vi "LTVUnicycleCtrl_Execute.vi"(4 "dT Sec":dbl=0.02, 5 "LTV_Unicycle_Ctrl_Model":T2={"Max linear ctrl effort M/S"=1.0, "Max angular ctrl effort Rad/S"=2.0, "Max Heading Meas Tol Rad"=0.2, "Max X Pos Meas Tol M"=0.0625, "Max Y Pos Meas Tol M"=0.125, "Max Linear Vel M/S"=9.0} {"Max Linear Vel M/S" format="%#_13g"; "Max Y Pos Meas Tol M" format="%#_13g"; "Max X Pos Meas Tol M" format="%#_13g"; "Max Heading Meas Tol Rad" format="%#_13g"; "Max angular ctrl effort Rad/S" format="%#_13g"; "Max linear ctrl effort M/S" format="%#_13g"}, 6 "Enabled":bool=TRUE, 7 "LTV_Unicycle_Ctrl_Tolerance":T1={"Max Heading Tolerance Rad"=1.0, "Max X Tolerance M"=2.0, "Max Y Tolerance M"=0.2} {"Max Y Tolerance M" format="%#_13g"; "Max X Tolerance M" format="%#_13g"; "Max Heading Tolerance Rad" format="%#_13g"}, 8 "CurrentPose":T4={"TRANSLATION"={"X"=0.0, "Y"=0.0}, "ROTATION"={"VALUE"=0.0, "COS"=1.0, "SIN"=0.0}} {"ROTATION"."SIN" format="%13.4f"; "ROTATION"."COS" format="%13.4f"; "ROTATION"."VALUE" format="%13.4f"; "TRANSLATION"."Y" format="%14.3f"; "TRANSLATION"."X" format="%14.3f"}, 9 "RefAngularVelocity":dbl, 10 "RefLinearVelocity":dbl, 11 "RefPose":T4={"TRANSLATION"={"X"=0.0, "Y"=0.0}, "ROTATION"={"VALUE"=0.0, "COS"=1.0, "SIN"=0.0}} {"ROTATION"."SIN" format="%13.4f"; "ROTATION"."COS" format="%13.4f"; "ROTATION"."VALUE" format="%13.4f"; "TRANSLATION"."Y" format="%14.3f"; "TRANSLATION"."X" format="%14.3f"}) -> (0 "Error":bool, 1 "out LTV_UNICYCLE_CONTROLLER":T7={"States"=0, "Inputs"=0, "PoseError"={"TRANSLATION"={"X"=0.0, "Y"=0.0}, "ROTATION"={"VALUE"=0.0, "COS"=1.0, "SIN"=0.0}}, "PoseTolerance"={"TRANSLATION"={"X"=0.0, "Y"=0.0}, "ROTATION"={"VALUE"=0.0, "COS"=1.0, "SIN"=0.0}}, "Dt"=0.02, "Enabled"=FALSE, "LQR_K_Table"={"Table Xs"=[], "Table Ys"=[], "MinX"=0.0, "MaxX"=0.0, "ItemCount"=0, "Rows"=0, "Columns"=0}} {"PoseTolerance"."ROTATION"."SIN" format="%13.4f"; "PoseTolerance"."ROTATION"."COS" format="%13.4f"; "PoseTolerance"."ROTATION"."VALUE" format="%13.4f"; "PoseTolerance"."TRANSLATION"."Y" format="%14.3f"; "PoseTolerance"."TRANSLATION"."X" format="%14.3f"; "PoseError"."ROTATION"."SIN" format="%13.4f"; "PoseError"."ROTATION"."COS" format="%13.4f"; "PoseError"."ROTATION"."VALUE" format="%13.4f"; "PoseError"."TRANSLATION"."Y" format="%14.3f"; "PoseError"."TRANSLATION"."X" format="%14.3f"}, 2 "At Reference":bool, 3 "ChassisSpeeds":T3 {"vOmega" format="%10.3f"; "vY" format="%10.3f"; "vX" format="%10.3f"})   [LabVIEW 2019, in "Trajectory_Library.lvlib"]
doc: "The linear time-varying unicycle controller has a similar form to the LQR, but the model used to compute the controller gain is the nonlinear model linearized around the drivetrain's current state.\n\nThis LabVIEW single call function creates and executes the LTV Unicycle controller. \n\n\nInputs:\n - LTVUnicycleCtrl Model -- cluster -- Packed data used to construct the LTV Unicycle control system.\n - LTVUnicycleCtrl Tol -- cluster -- Packed data used to define the tolerance LTV Unicycle control system.\n - Ref Pose -- Pose2d -- The desired pose setpoint. (Meters, Radians)\n - Ref Linear Velocity -- double -- The desired linear velocity (Meters/sec)\n - Ref Angular Velocity -- double -- The desired angular velocity (Radians/sec)\n - Current Pose -- Pose2d -- The current pose. (Meters, Radians)\n - Enabled -- boolean -- If TRUE use closed loop control to calculate desired chassis speeds. If FALSE, outputs the reference speeds directly.\n - dt Sec -- double -- Update time (default: 0.02)\n\nOutputs:\n - Chassis Speed -- chassis speed -- Chassis Speed Demand\n - At Reference -- boolean -- If TRUE, the current position is within the tolerance.\n - Error -- boolean -- If TRUE, an error occured.\n - out LTV UnicycleCtrl -- cluster -- Internal data structure."
uses:
  Trajectory_Library.lvlib
  TypeDef/LTV_UNICYCLE_CONTROLLER.ctl
  TypeDef/POSE2D.ctl
  TypeDef/TRANSLATION2D.ctl
  TypeDef/ROTATION2D.ctl
  TypeDef/FUNCTION_GENERATOR_MATRIX.ctl
  TypeDef/CHASSIS_SPEEDS.ctl
  TypeDef/LTV_UNICYCLE_CONTROLLER_MODEL_PARAMS.CTL
  TypeDef/LTV_UNICYCLE_CONTROLLER_TOLERANCE.CTL
  Rotation2d_CreateAngle.vi
  Translation2d_Create.vi
  MatBuilder_Create.vi
  Pose2d_getXYAngle.vi
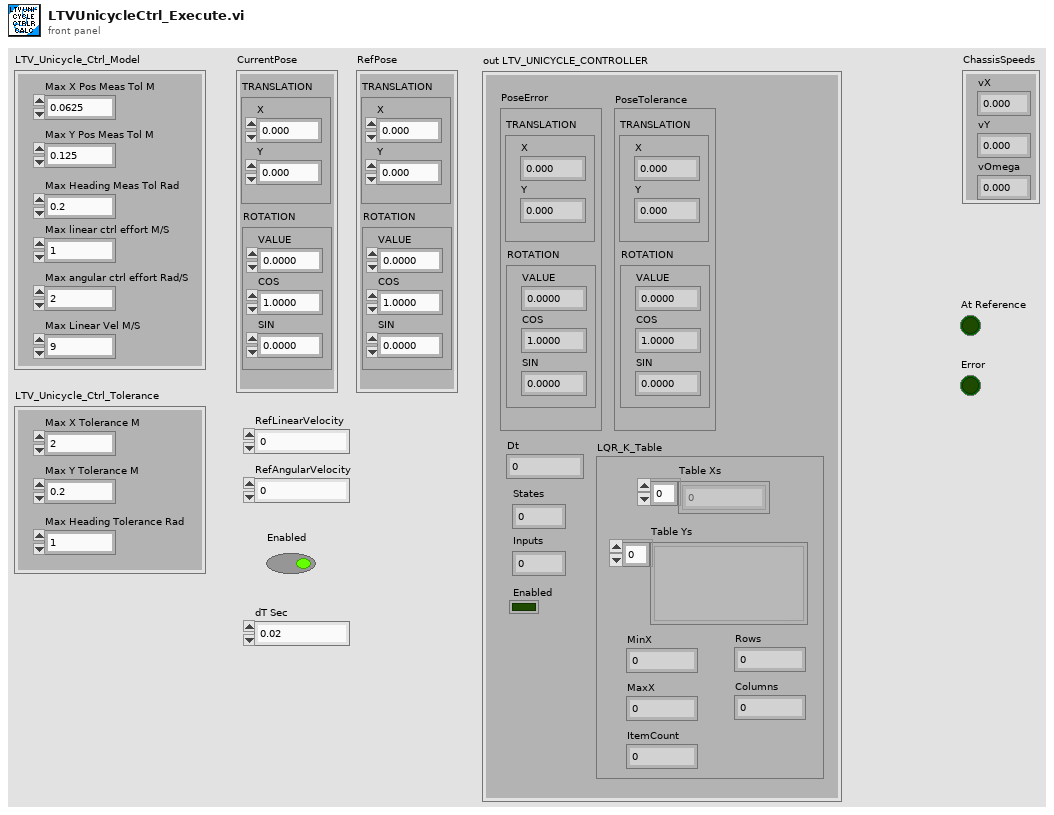
[diagram p1: front panel]
types:
  T1 = typedef "Trajectory_Library.lvlib/LTV_UNICYCLE_CONTROLLER_TOLERANCE.CTL" = cluster{"Max Heading Tolerance Rad":dbl, "Max X Tolerance M":dbl, "Max Y Tolerance M":dbl}
  T2 = typedef "Trajectory_Library.lvlib/LTV_UNICYCLE_CONTROLLER_MODEL_PARAMS.CTL" = cluster{"Max linear ctrl effort M/S":dbl, "Max angular ctrl effort Rad/S":dbl, "Max Heading Meas Tol Rad":dbl, "Max X Pos Meas Tol M":dbl, "Max Y Pos Meas Tol M":dbl, "Max Linear Vel M/S":dbl}
  T3 = typedef "Trajectory_Library.lvlib/CHASSIS_SPEEDS.ctl" = cluster{"vX":dbl, "vY":dbl, "vOmega":dbl}
  T4 = typedef "Trajectory_Library.lvlib/POSE2D.ctl" = cluster{"TRANSLATION":T5, "ROTATION":T6}
  T5 = typedef "Trajectory_Library.lvlib/TRANSLATION2D.ctl" = cluster{"X":dbl, "Y":dbl}
  T6 = typedef "Trajectory_Library.lvlib/ROTATION2D.ctl" = cluster{"VALUE":dbl, "COS":dbl, "SIN":dbl}
  T7 = typedef "Trajectory_Library.lvlib/LTV_UNICYCLE_CONTROLLER.ctl" = cluster{"States":i32, "Inputs":i32, "PoseError":T4, "PoseTolerance":T4, "Dt":dbl, "Enabled":bool, "LQR_K_Table":T8}
  T8 = typedef "Trajectory_Library.lvlib/FUNCTION_GENERATOR_MATRIX.ctl" = cluster{"Table Xs":dbl[], "Table Ys":variant[], "MinX":dbl, "MaxX":dbl, "ItemCount":i32, "Rows":i32, "Columns":i32}
  T9 = typedef "NI_Matrix.lvlib/RealMatrix.ctl" = dbl[][]
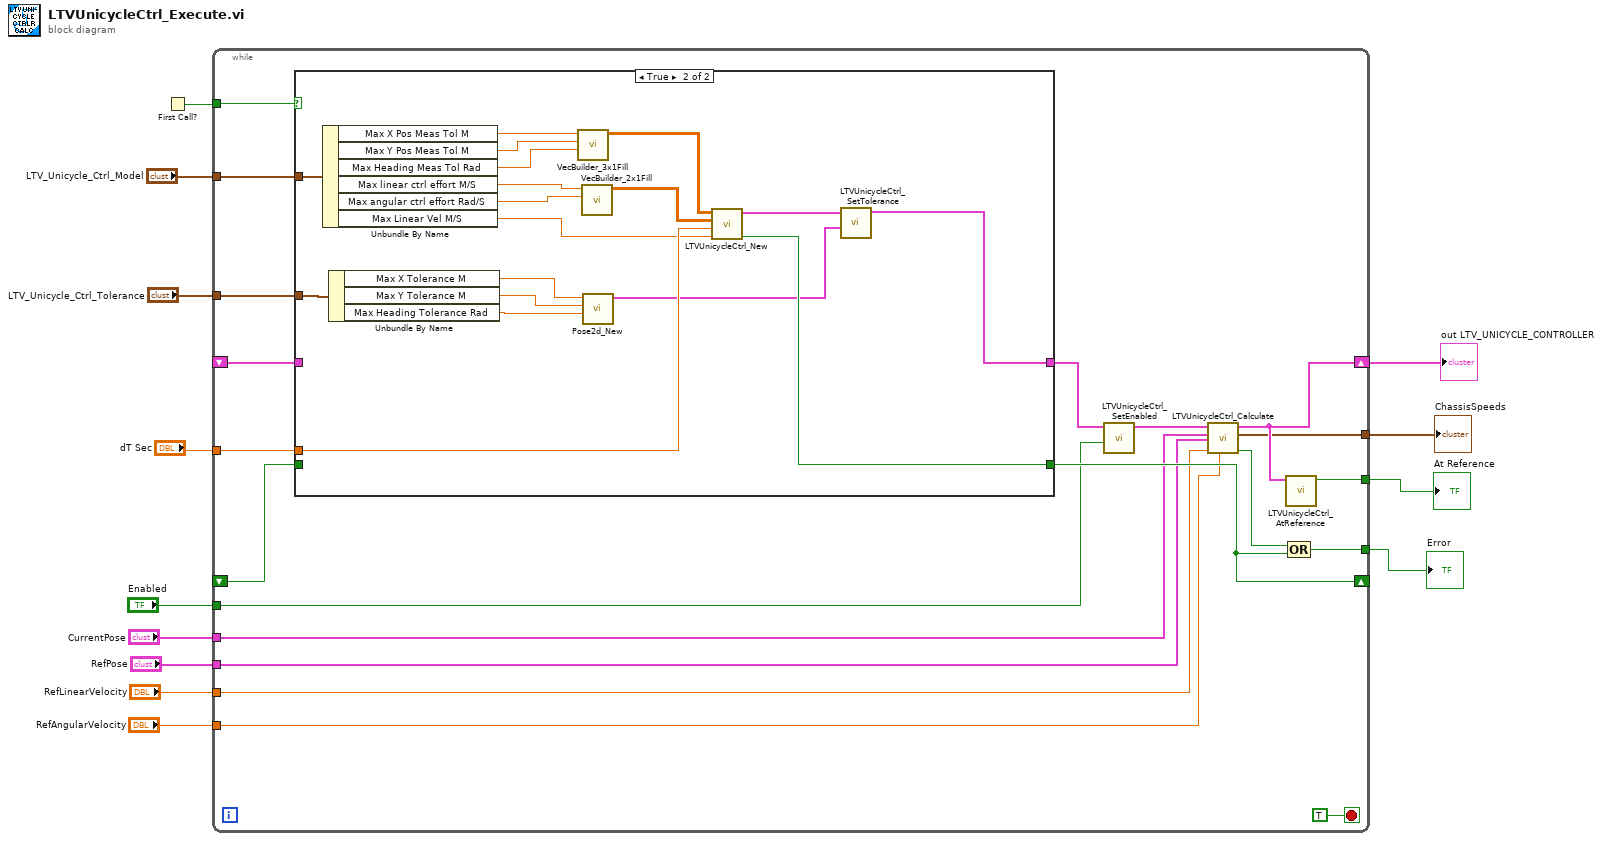
[diagram p0: block diagram]
diagram:
  n1 = First Call?() -> (First Call?: T/F=w9:bool)
  n2 = while {
    shift-right: [w33] -> w10
    shift-left: _ -> [w26]
    tunnel: [w31] -> w13
    tunnel: [w30] -> w12
    tunnel: [w28] -> w11
    tunnel: w9 -> [w25]
    shift-right: [w24] -> _
    shift-left: _ -> [w23]
    tunnel: "Enabled" -> [w22]
    tunnel: "CurrentPose" -> [w21]
    tunnel: "RefPose" -> [w20]
    tunnel: "RefLinearVelocity" -> [w19]
    tunnel: "RefAngularVelocity" -> [w18]
    tunnel: "dT Sec" -> [w17]
    tunnel: "LTV_Unicycle_Ctrl_Model" -> [w15]
    tunnel: "LTV_Unicycle_Ctrl_Tolerance" -> [w14]
    stop <- TRUE stop-if-true
    n3 = case shown="True" w25 {
      tunnel: [w35 w53] -> w27
      tunnel: w26 -> [w35 _]
      tunnel: [w34 w51] -> w24
      tunnel: w23 -> [w34 _]
      tunnel: w17 -> [_ w50]
      tunnel: w15 -> [_ w49]
      tunnel: w14 -> [_ w39]
      frame False {
      }
      frame True {
        n4 = Unbundle By Name(w49) -> ("Max X Pos Meas Tol M"=w46:dbl, "Max Y Pos Meas Tol M"=w45:dbl, "Max Heading Meas Tol Rad"=w44:dbl, "Max linear ctrl effort M/S"=w43:dbl, "Max angular ctrl effort Rad/S"=w42:dbl, "Max Linear Vel M/S"=w41:dbl)
        n5 = Unbundle By Name(w39) -> ("Max X Tolerance M"=w38:dbl, "Max Y Tolerance M"=w37:dbl, "Max Heading Tolerance Rad"=w36:dbl)
        n6 = call "VecBuilder_3x1Fill.vi"("R2"=w44, "R1"=w45, "R0"=w46) -> ("output matrix"=w48:T9)  [unwired: 8 in]
        n7 = call "VecBuilder_2x1Fill.vi"("R1"=w42, "R0"=w43) -> ("output matrix"=w47:T9)  [unwired: 9 in]
        n8 = call "Pose2d_New.vi"("Heading"=w36, "Y"=w37, "X"=w38) -> ("out POSe"=w40:T4)  [unwired: 8 in]
        n9 = call "LTVUnicycleCtrl_New.vi"("Max Velocity"=w41, "dT"=w50, "RELMS"=w47, "QELMS"=w48) -> ("Error"=w51:bool, "LTV_UNICYCLE_CONTROLLER"=w52:T7)  [unwired: 6 in]
        n10 = call "LTVUnicycleCtrl_SetTolerance.vi"("Tolerance"=w40, "in LTV_UNICYCLE_CONTROLLER"=w52) -> ("out LTV_UNICYCLE_CONTROLLER"=w53:T7)  [unwired: 9 in]
      }
    }
    n11 = call "LTVUnicycleCtrl_SetEnabled.vi"("Enabled"=w22, "in LTV_UNICYCLE_CONTROLLER"=w27) -> ("out LTV_UNICYCLE_CONTROLLER"=w32:T7)  [unwired: 9 in]
    n12 = call "LTVUnicycleCtrl_Calculate.vi"("RefAngularVelocity"=w18, "RefLinearVelocity"=w19, "RefPose"=w20, "CurrentPose"=w21, "in LTV_UNICYCLE_CONTROLLER"=w32) -> ("Error"=w29:bool, "ChassisSpeeds"=w31:T3, "out LTV_UNICYCLE_CONTROLLER"=w33:T7)  [unwired: 4 in]
    n13 = call "LTVUnicycleCtrl_AtReference.vi"("LTV_UNICYCLE_CONTROLLER"=w33) -> ("At Reference"=w30:bool)  [unwired: 10 in]
    n14 = Compound Arithmetic op=OR(w29, w24) -> (w28:bool)
  }
  "out LTV_UNICYCLE_CONTROLLER" <- w10
  "Error" <- w11
  "ChassisSpeeds" <- w13
  "At Reference" <- w12
